vi "String+Case Structure Coin Toss.vi"() -> ()   [LabVIEW 2019]
uses:
  <vilib>/numeric/Random Number (Range) U64.vi
  <vilib>/numeric/sub_Random U32.vi
panel:
  out "Head or Tail?":string
  # "Challenge:\nWrite a program to flip a coin, Each time you run the program, HEAD or TAIL is displayed randomly with equal probability."
  # "Try it: Run the program."
  # "You will probably need:\nRandom number generator, string, case structure"
  # "Open the block diagram to see a possible solution."
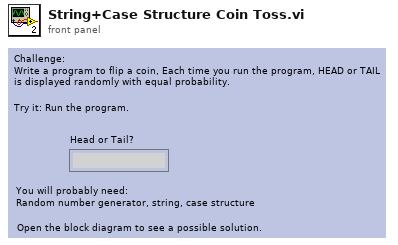
[diagram p1: front panel]
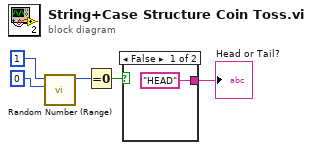
[diagram p0: block diagram]
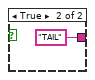
[diagram p2: hidden frame]
diagram:
  n1 = call-poly <vilib>:"Random Number (Range).vi"("lower bound (0)"=u64 0 ("upper bound (100)"), "upper bound (100)"=u64 1) -> ("number"=w3:u64)  [unwired: 9 in]
  n2 = Equal To 0?(x=w3) -> (x = 0?=w2:bool)
  n3 = case shown="False" w2 {
    tunnel: ["HEAD" "TAIL"] -> w1
    frame False {
    }
    frame True {
    }
  }
  "Head or Tail?" <- w1
